vi "Pruebas_basura.vi"() -> ()   [LabVIEW 2020]
uses:
  <vilib>/vision/NI_Vision_Development_Module.lvlib
panel:
  out "Analisis frontal 5":T1(plugin-control)
  out "Analisis frontal 3":T1(plugin-control)
  out "Analisis frontal 2":T1(plugin-control)
  in  "Replace Value":sgl=1.0 format="%.2f"
  in  "Keep/Replace Value (Replace)":bool=TRUE
  in  "Range":cluster{"Lower value":sgl, "Upper value":sgl}={"Lower value"=128.0, "Upper value"=255.0} {"Upper value" format="%.2f"; "Lower value" format="%.2f"}
  in  "new picture 2":picture
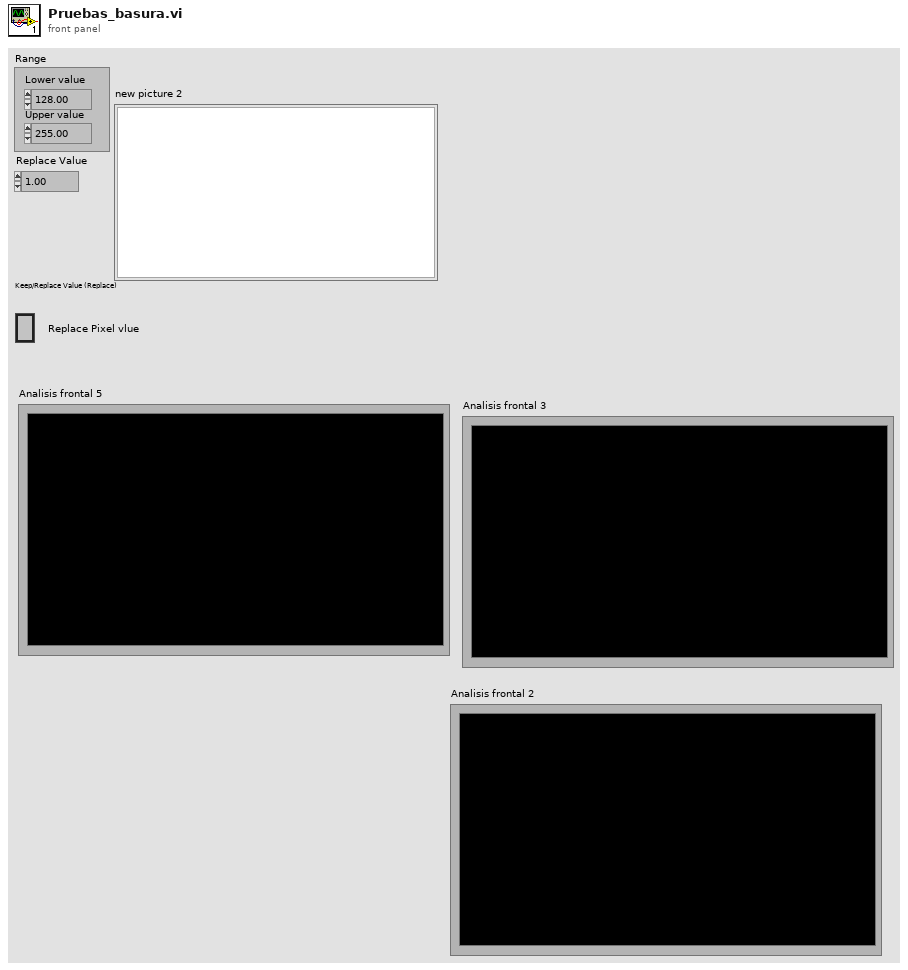
[diagram p1: front panel]
types:
  T1 = typedef "IMAQ Image.ctl" = refnum<image>
  T2 = typedef "Image Type" = u32
  T3 = typedef "imagedata.ctl" = cluster{"image type":i32, "image depth":i32, "image":u8[], "mask":u8[], "colors":u32[], "Rectangle":cluster{"left":i16, "top":i16, "right":i16, "bottom":i16}}
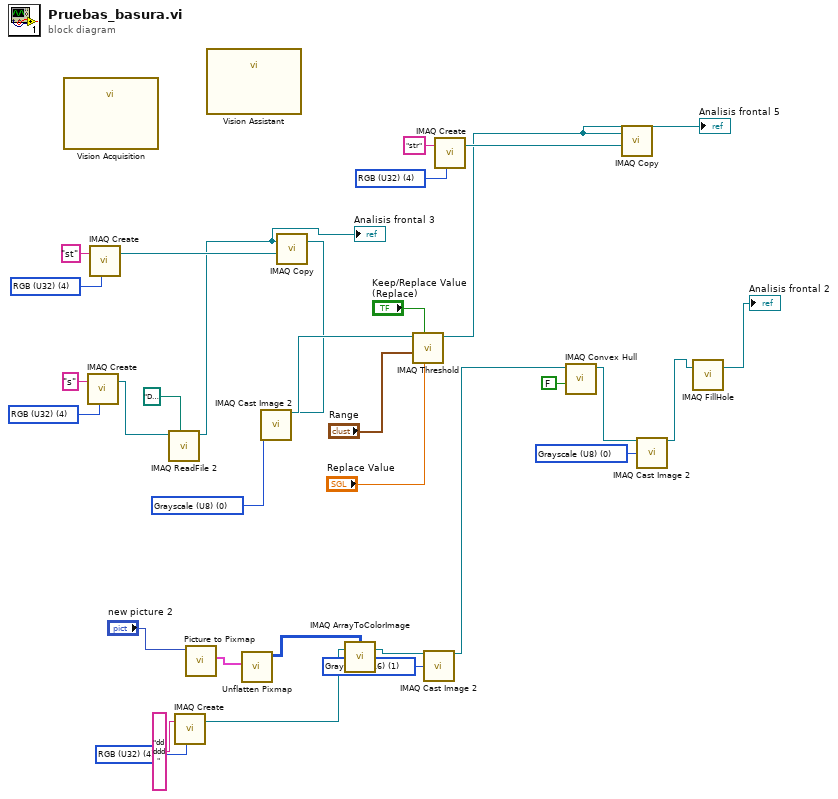
[diagram p0: block diagram]
diagram:
  w1 = T2 0 items=["Grayscale (U8)", "Grayscale (I16)", "Grayscale (SGL)", "Complex (CSG)", "RGB (U32)", "HSL (U32)", "RGB (U64)", "Grayscale (U16)"] ("Image Type")
  w6 = T2 1 items=["Grayscale (U8)", "Grayscale (I16)", "Grayscale (SGL)", "Complex (CSG)", "RGB (U32)", "HSL (U32)", "RGB (U64)", "Grayscale (U16)"] ("Image Type")
  w10 = T2 4 items=["Grayscale (U8)", "Grayscale (I16)", "Grayscale (SGL)", "Complex (CSG)", "RGB (U32)", "HSL (U32)", "RGB (U64)", "Grayscale (U16)"] ("Image Type")
  w19 = T2 4 items=["Grayscale (U8)", "Grayscale (I16)", "Grayscale (SGL)", "Complex (CSG)", "RGB (U32)", "HSL (U32)", "RGB (U64)", "Grayscale (U16)"] ("Image Type")
  w20 = T2 4 items=["Grayscale (U8)", "Grayscale (I16)", "Grayscale (SGL)", "Complex (CSG)", "RGB (U32)", "HSL (U32)", "RGB (U64)", "Grayscale (U16)"] ("Image Type")
  w24 = T2 0 items=["Grayscale (U8)", "Grayscale (I16)", "Grayscale (SGL)", "Complex (CSG)", "RGB (U32)", "HSL (U32)", "RGB (U64)", "Grayscale (U16)"] ("Image Type")
  w28 = T2 4 items=["Grayscale (U8)", "Grayscale (I16)", "Grayscale (SGL)", "Complex (CSG)", "RGB (U32)", "HSL (U32)", "RGB (U64)", "Grayscale (U16)"] ("Image Type")
  n1 = call "Vision Acquisition"() -> ()  [unwired: 12 in]
  n2 = call "IMAQ Create"("Image Name"="s", "Image Type"=w28) -> ("New Image"=w26:T1)  [unwired: 3 in, 1 out]
  n3 = call "IMAQ Create"("Image Name"="st", "Image Type"=w20) -> ("New Image"=w21:T1)  [unwired: 3 in, 1 out]
  n4 = call "IMAQ ReadFile 2"("File Path"=path "D:/lzggz/Pictures/Camera Roll/1.jpg", "Image"=w26) -> ("Image Out"=w14:T1)  [unwired: 5 in, 4 out]
  "Analisis frontal 3" <- w14
  n5 = call "IMAQ Create"("Image Name"="ddddd", "Image Type"=w10) -> ("New Image"=w8:T1)  [unwired: 3 in, 1 out]
  n6 = call <vilib>:"Picture to Pixmap.vi"("picture"="new picture 2") -> ("image data"=w12:T3)  [unwired: 9 in, 1 out]
  n7 = call "Vision Assistant"() -> ()  [unwired: 26 in, 2 out]
  n8 = call <vilib>:"Unflatten Pixmap.vi"("image data"=w12) -> ("24-bit pixmap"=w11:u32[][])  [unwired: 4 in, 6 out]
  n9 = call "IMAQ Copy"("Image Dst"=w21, "Image Src"=w14) -> ("Image Dst Out"=w15:T1)  [unwired: 4 in, 1 out]
  n10 = call "IMAQ Cast Image 2"("Image Src"=w15, "Image Type"=w24) -> ("Image Dst Out"=w25:T1)  [unwired: 12 in, 1 out]
  n11 = call "IMAQ ArrayToColorImage"("Image Pixels (U32)"=w11, "Image"=w8) -> ("Image Out"=w7:T1)  [unwired: 3 in, 1 out]
  n12 = call "IMAQ Threshold"("Replace Value"="Replace Value", "Keep/Replace Value (Replace)"="Keep/Replace Value (Replace)", "Range"="Range", "Image Src"=w25) -> ("Image Dst Out"=w16:T1)  [unwired: 6 in, 1 out]
  "Analisis frontal 5" <- w16
  n13 = call "IMAQ Cast Image 2"("Image Src"=w7, "Image Type"=w6) -> ("Image Dst Out"=w5:T1)  [unwired: 12 in, 1 out]
  n14 = call "IMAQ Create"("Image Name"="str", "Image Type"=w19) -> ("New Image"=w18:T1)  [unwired: 3 in, 1 out]
  n15 = call "IMAQ Convex Hull"("Connectivity 4/8 (8)"=FALSE, "Image Src"=w5) -> ("Image Dst Out"=w3:T1)  [unwired: 8 in, 1 out]
  n16 = call "IMAQ Copy"("Image Dst"=w18, "Image Src"=w16) -> ()  [unwired: 4 in, 2 out]
  n17 = call "IMAQ Cast Image 2"("Image Src"=w3, "Image Type"=w1) -> ("Image Dst Out"=w2:T1)  [unwired: 12 in, 1 out]
  n18 = call "IMAQ FillHole"("Image Src"=w2) -> ("Image Dst Out"=→"Analisis frontal 2":T1)  [unwired: 5 in, 1 out]
